vi "LVClass_HasoData ctor from file.vi"(0 "HasoData (const)":refnum<class "HasoData.lvclass">, 5 "HAS file path":path, 11 "error in (no error)":errorcluster) -> (4 "HasoData (new)":refnum<class "HasoData.lvclass">, 15 "error out":errorcluster)   [LabVIEW 2020, in "HasoData.lvclass"]
doc: "HasoData constructor from a .has file. If file opening fails, an exception is\nthrown.\n\n--------------------------------------------------------------------------------\n\n<B>HasoDataIn </B> : Constant Pointer to HasoData object.\n<B>HasoDataOut </B> : Constant Pointer to HasoData object.\n<B>has_file_path </B> : Absolute path to .has file.\n<B>ErrorIn </B> : Error\n<B>ErrorOut </B> : Error\n\n--------------------------------------------------------------------------------"
uses:
  HasoData.lvclass
  Controls/Handle creation.ctl
  HasoData.lvclass/HasoData.ctl
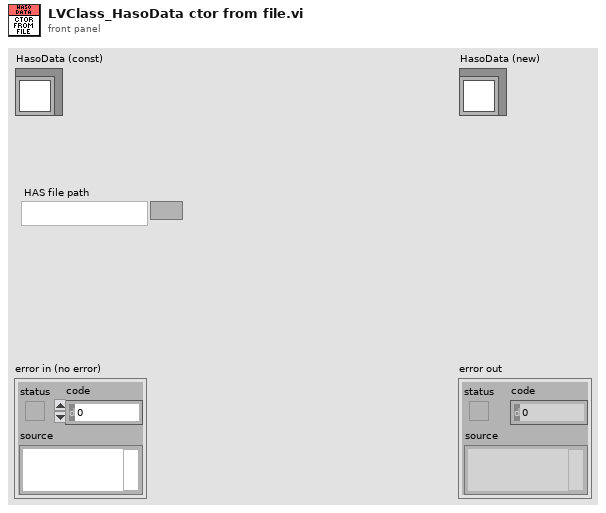
[diagram p1: front panel]
types:
  T1 = typedef "Handle creation.ctl" = enum16{"By ctor", "By write function"}
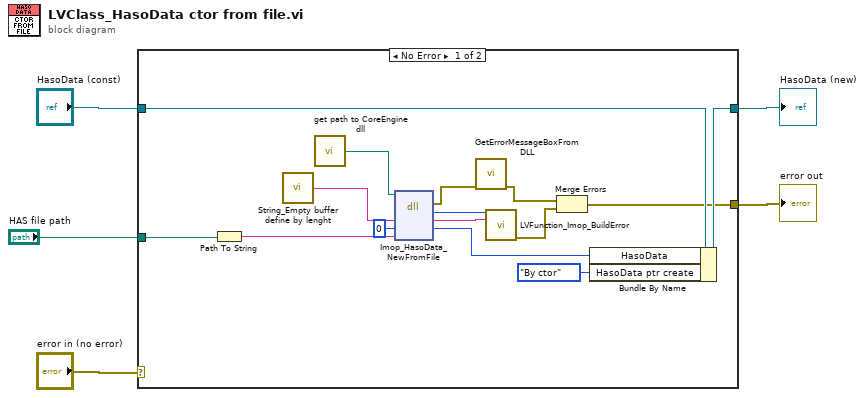
[diagram p0: block diagram]
diagram:
  n1 = case shown="No Error" "error in (no error)" {
    selector: "error in (no error)" -> [_ w22]
    tunnel: [w6 w22] -> w2
    tunnel: [w15 w21] -> w3
    tunnel: "HasoData (const)" -> [w16 w21]
    tunnel: "HAS file path" -> [w10 _]
    frame No Error {
      n2 = Path To String(path=w10) -> (string=w9:string)
      n3 = call "String_Empty buffer define by lenght.vi"() -> ("Empty buffer"=w14:string)  [unwired: 1 in]
      n4 = call "get path to CoreEngine dll.vi"() -> ("path to wavekit library"=w13:path)  [unwired: 14 in, 1 out]
      n5 = dll-call lib="D:/soft/HASO_v3/SVN_trunk/ImOpCoreEngine4_LV2011/DLLs/c_interface_vc100.dll" fn="Imop_HasoData_NewFromFile"(path in=w13, "message"=w14, "objet"=0, "chemin_config"=w9) -> (error out=w12:errorcluster, "return type"=w19:i32, "message"=w18:string, "objet"=w17:i64)  [unwired: 3 in, 1 out]
      n6 = call "GetErrorMessageBoxFromDLL.vi"("error IN"=w12) -> ("error OUT"=w8:errorcluster)  [unwired: 10 in]
      n7 = call "LVFunction_Imop_BuildError.vi"("code"=w19, "String to Prepend to source (\"\")"=w18) -> ("error out"=w7:errorcluster)  [unwired: 13 in]
      n8 = Merge Errors(w8, w7) -> (w6:errorcluster)
      n9 = Bundle By Name(cluster=w16, "HasoData"=w17, "HasoData ptr create"=Handle_creation."By ctor") -> (w15:refnum<class "HasoData.lvclass">)
    }
    frame Error {
    }
  }
  "error out" <- w2
  "HasoData (new)" <- w3
